vi "Process Controller.vi"() -> ()   [LabVIEW 2015]
doc: "Uses the next generation of Stamp control boxes that have the ability to control pump direction. \n\nAutomatically saves configuration changes to Process Controller.pcm in the same folder as the application.\nKeeps track of whether the program was shutdown correctly with a boolean in the ini file. If the software doesn't shutdown correctly it will automatically resume where it left off (same configuration and same state) as when it was shutdown.\nSaves state name in the state log.\n**********************************\nNo longer reloads setpoint code when not necessary to prevent losing data stored in external code.\nNo longer updates sensor buffer if data wasn't received.\nThe calculated values of setpoints can be viewed \"live\" within the rule editor. This update also adds fields for labeling the output controls. This software can not open the rule files created with previous versions."
uses:
  Plant mode.ctl
  Plant state.ctl
  DAQ configuration/Sensor buffer command.ctl
  file/file action.ctl
  toolbar icons/log data.ctl
  Stamp/calibration commands.ctl
  data status.ctl
  Stamp/stamp command.ctl
  read-write.ctl
  ini interface.ctl
  default or user select.ctl
  toolbar icons/Data Source.ctl
  toolbar icons/peristaltic pump.ctl
  toolbar icons/calibrator.ctl
  toolbar icons/edit rules.ctl
  toolbar icons/Save configuration.ctl
  toolbar icons/open configuration.ctl
  Plant method.ctl
  operator info.ctl
  switch and fraction.ctl
  TCP DAQ/Sensor data.ctl
  DAQ configuration/sensor cluster.ctl
  toolbar icons/file comment.ctl
  toolbar icons/help.ctl
  toolbar icons/Export pcm.ctl
panel:
  in  "Help Button":T1
  out "auto datalogref":refnum<file>
  out "user datalog ref":refnum<file>
  out "TCP ID":refnum<k5>
  in  "Tab Control":T2(tab)=enum."Plant Operation"
  in  "export pcm":T3
  out "data server":string="128.84.245.227"
  out "sensor range error":bool
  in  "Serial Port":refnum<visa-resource-name>="COM1"
  out "Stamp com Failure":bool
  in  "Peristaltic Pump":T4
  in  "Data Source":T5 caption="OK Button"
  in  "Quit":bool
  out "data rate (Hz)":dbl
  out "Datalog File Failure":bool
  in  "Calibrate Sensors":T6
  in  "Edit Rules":T7
  in  "Save":T8
  in  "open":T9
  in  "Process Method":T10={"Operator information"=[], "data log interval"=5, "data loop interval"=20, "Datalog directory path"=path "", "graph update interval"=1.0, "history length"=1000, "Control Logic file path"=path "C:/Documents and Settings/mw24/Desktop/rules.rul", "Sensor Configuration file path"=path "", "HMI VI path"=path "", "HMI data smooth"=0.1} {"HMI data smooth" min=0.01 format="%.2f"; "history length" min=1; "graph update interval" min=0.001 format="%.2f"; "data log interval" min=1}
  out "output descriptions 2":string[][](array[string])
  out "controls 2":T12 {"fractional duty" format="%#_3g"}
  out "Data Status":T13
  out "output descriptions":string[][](array[string])
  in  "Data log interval":sgl=5.0 min=0.01 step=0.01
  in  "Log Data":T14
  in  "File Comment":T15
  out "controls":T12 {"fractional duty" format="%#_3g"}
  in  "Operator Selected State":u16(ring)=1 items=["OFF"]
  out "Elapsed time in current state":dbl format="%.2f"
  out "Process State":u16(ring)=1 items=["OFF"]
  in  "Mode of Operation":T16=enum."Automatic Operation"
  in  "Clear graph":bool
  out "Sensor Data":T17 {"Sensor array"."scaled" format="%.2f"; "Sensor array"."voltage" format="%.4f"; "Time" format="%<%I:%M:%S%2u %p\n%m/%d/%Y>T"}
  out "state graph":cluster{dbl[], dbl[]}(graph)
  in  "sensor to plot":u16(ring) items=["floc interface ()"]
  out "Sensor graph":cluster{dbl[], dbl[]}(graph)
  # "Method files (sensors, rules, calibrations)"
  # "Pump calibration"
  # "Data Source"
  # "Sensor configuration and calibration"
  # "Output communication with Stamp box"
  # "Output:\nstates rules setpoints, controls"
  # "s"
  # "pump off/on"
  # "0"
  # "1"
  # "pump cw/ccw"
  # "1"
  # "pump speed"
  # "2"
  # "pump off/on"
  # "3"
  # "2"
  # "pump cw/ccw"
  # "4"
  # "pump speed"
  # "5"
  # "pump off/on"
  # "6"
  # "3"
  # "pump cw/ccw"
  # "7"
  # "pump speed"
  # "8"
  # "pump off/on"
  # "9"
  # "4"
  # "pump cw/ccw"
  # "10"
  # "pump speed"
  # "11"
  # "pump off/on"
  # "12"
  # "5"
  # "pump cw/ccw"
  # "pump off/on"
  # "0"
  # "pump speed"
  # "pump cw/ccw"
  # "pump speed"
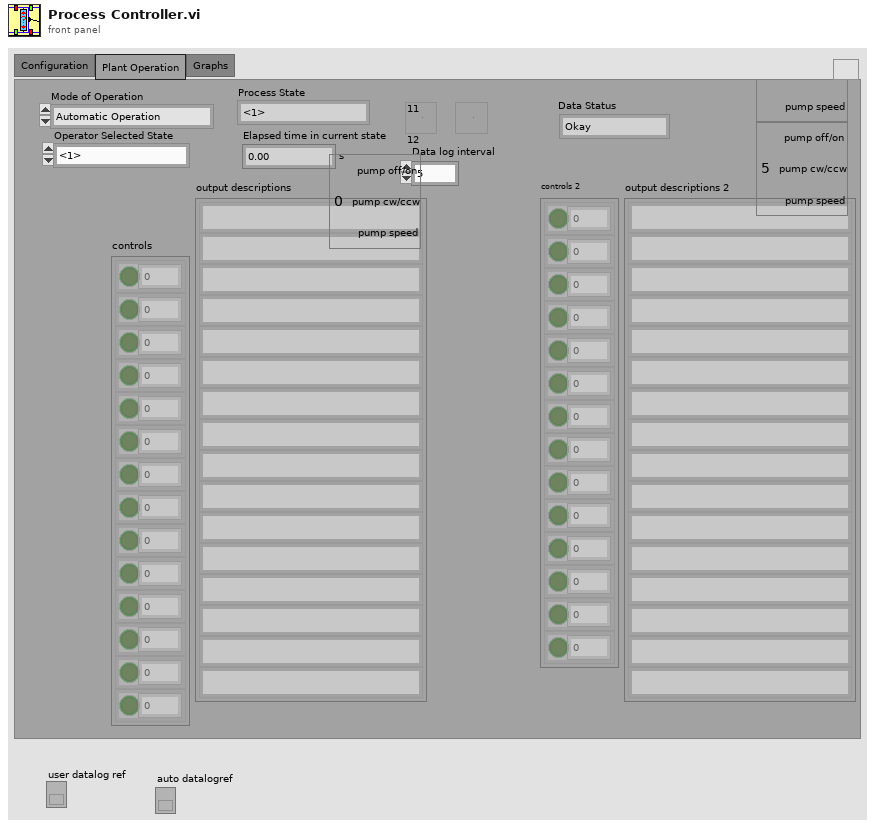
[diagram p1: front panel]
types:
  T1 = typedef "help.ctl" = bool
  T2 = enum32{"Configuration", "Plant Operation", "Graphs"}
  T3 = typedef "Export pcm.ctl" = bool
  T4 = typedef "peristaltic pump.ctl" = bool
  T5 = typedef "Data Source.ctl" = bool
  T6 = typedef "calibrator.ctl" = bool
  T7 = typedef "edit rules.ctl" = bool
  T8 = typedef "Save configuration.ctl" = bool
  T9 = typedef "open configuration.ctl" = bool
  T10 = typedef "Plant method.ctl" = cluster{"Operator information":T11, "data log interval":u32, "data loop interval":u32, "Datalog directory path":path, "graph update interval":sgl, "history length":u16, "Control Logic file path":path, "Sensor Configuration file path":path, "HMI VI path":path, "HMI data smooth":dbl}
  T11 = typedef "operator info.ctl" = cluster{"First name":string, "Last name":string, "NetID":string}[]
  T12 = typedef "switch and fraction.ctl" = cluster{"switch":bool, "fractional duty":dbl}[]
  T13 = typedef "data status.ctl" = enum16{"Okay", "Sensor Range error", "Server error"}
  T14 = typedef "log data.ctl" = bool
  T15 = typedef "file comment.ctl" = bool
  T16 = typedef "Plant mode.ctl" = enum16{"Manual Locked in State", "Automatic Operation"}
  T17 = typedef "Sensor data.ctl" = cluster{" Sensor array":T18[], "Time":dbl}
  T18 = typedef "sensor cluster.ctl" = cluster{"voltage":sgl, "scaled":sgl, "units":string, "Out of Range":bool}
  T19 = typedef "Sensor buffer command.ctl" = enum16{"read average", "read recent", "read all", "write", "set buffer size", "Read channel config", "Write channel config", "clear"}
  T20 = typedef "ini interface.ctl" = enum16{"dataserver list", "dataserver", "com port", "stamp model", "Local Daq"}
  T21 = typedef "read-write.ctl" = enum16{"read", "write"}
  T22 = typedef "calibration commands.ctl" = enum16{"Get ini Path", "Save default values", "Save new calibration", "Read calibration", "Apply calibration", "Read STAMP mb", "Write STAMP mb"}
  T23 = typedef "stamp command.ctl" = enum16{"Configure", "Write", "Off", "Close"}
  T24 = typedef "default or user select.ctl" = enum16{"Default", "User select"}
  T25 = typedef "file action.ctl" = enum16{"Save", "Open"}
  T26 = enum32{"invalid app kind", "Development System", "Run Time System", "Student Edition", "Embedded LabVIEW", "Evaluation", "Custom"}
  T27 = enum16{"open", "open or create", "create or replace", "create", "open (read only)"}
  T28 = typedef "Plant state.ctl" = u16
  T29 = typedef "calibration values.ctl" = cluster{"target 1":dbl[unit], "target 2":dbl[unit], "measured 1":dbl[unit], "measured 2":dbl[unit]}
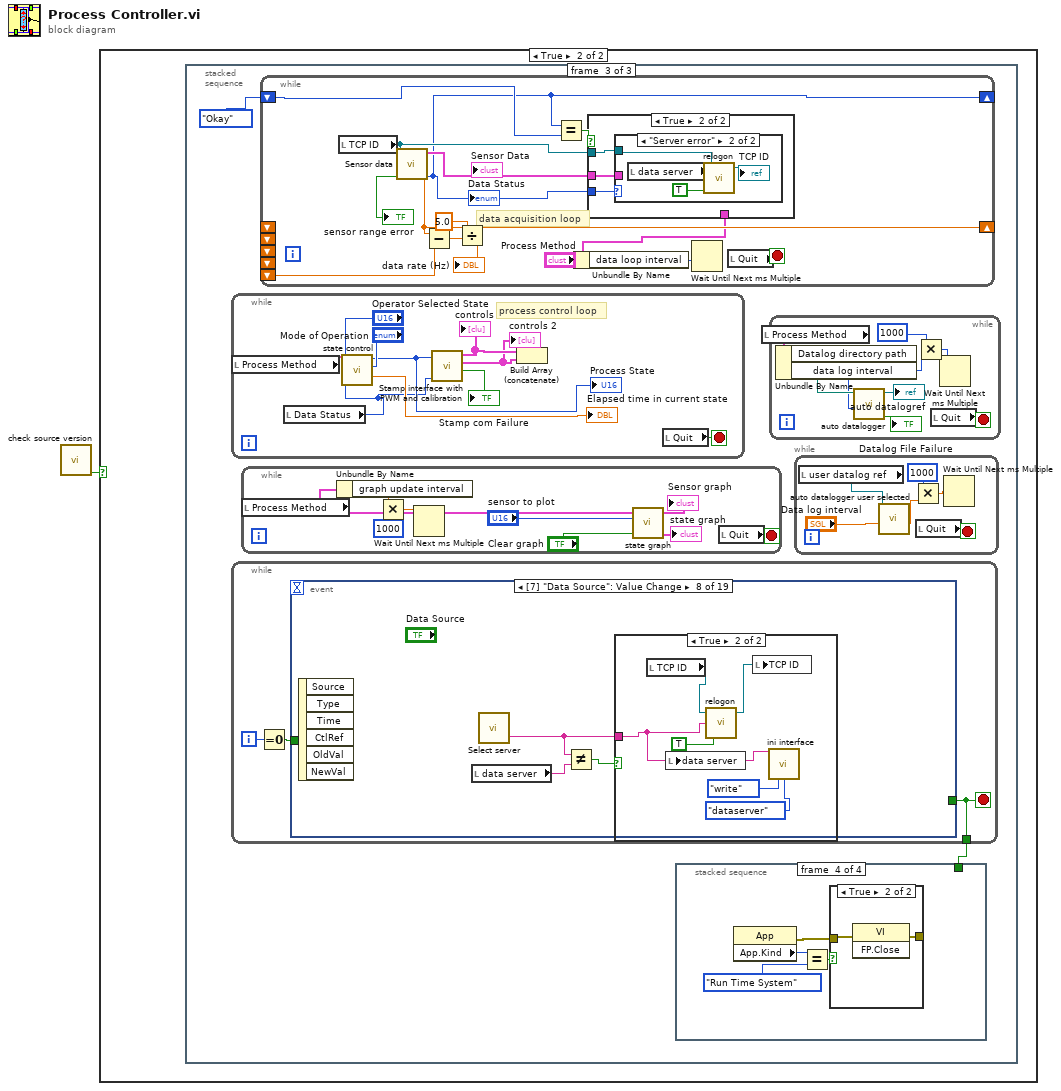
[diagram p0: block diagram]
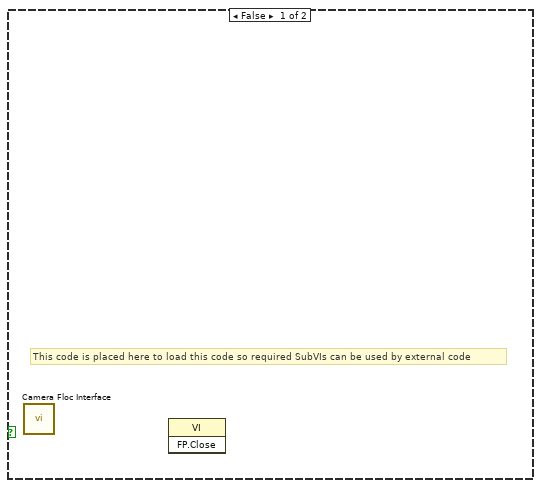
[diagram p2: hidden frame]
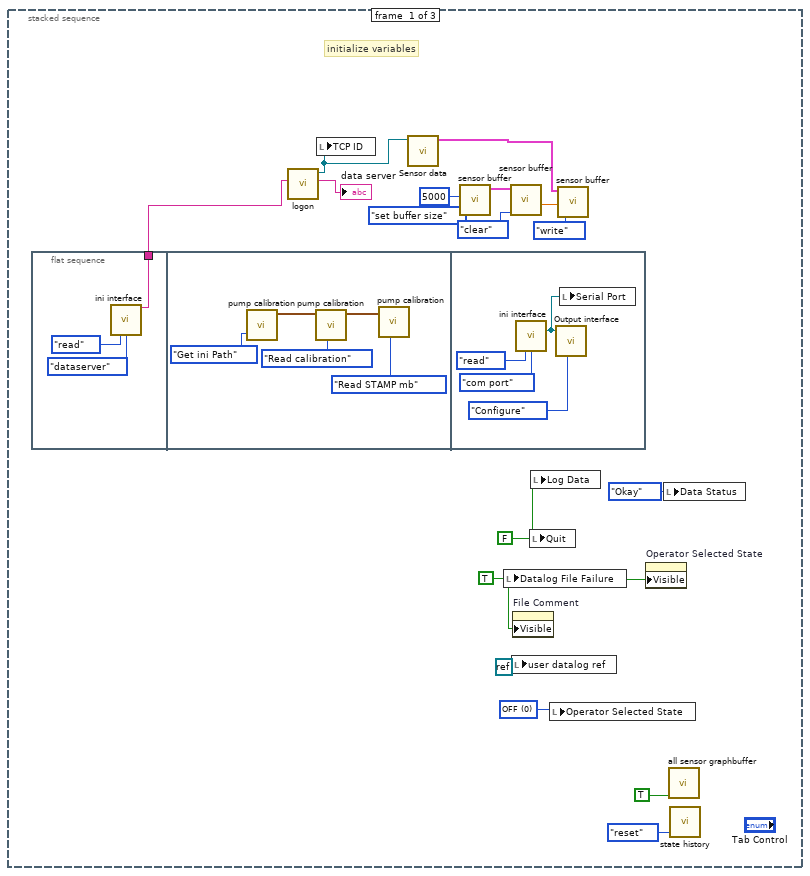
[diagram p3: hidden frame]
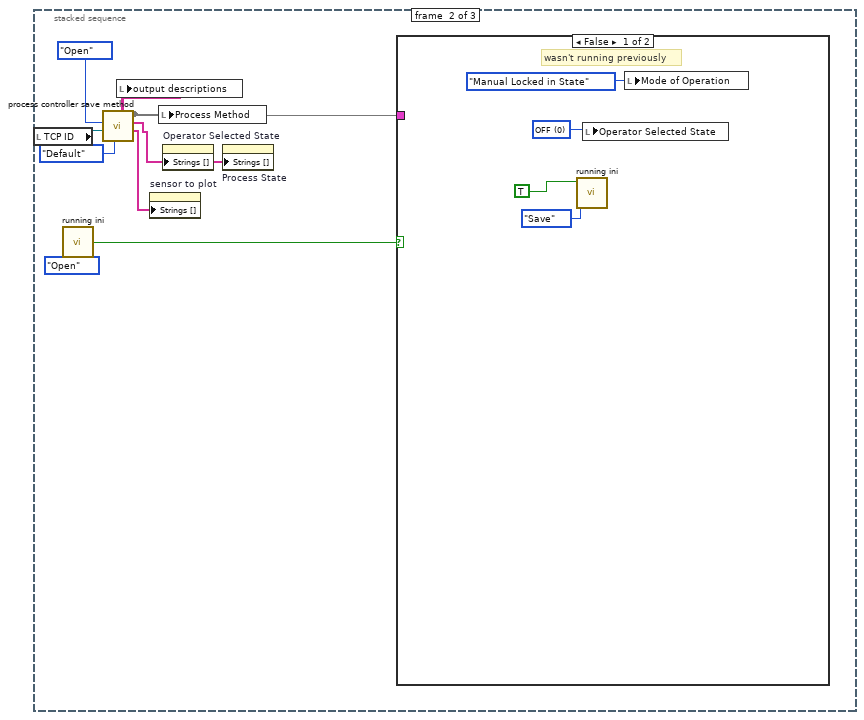
[diagram p4: hidden frame]
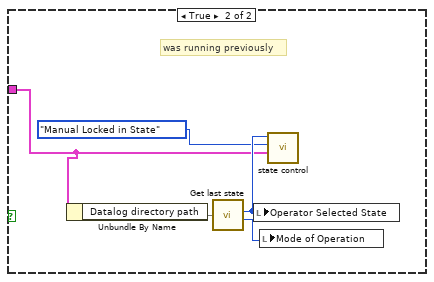
[diagram p5: hidden frame]
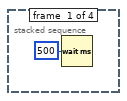
[diagram p6: hidden frame]
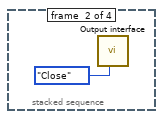
[diagram p7: hidden frame]
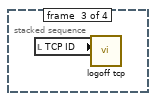
[diagram p8: hidden frame]
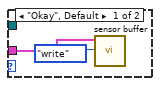
[diagram p11: hidden frame]
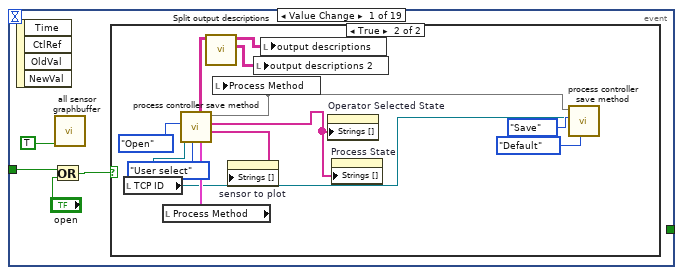
[diagram p12: hidden frame]
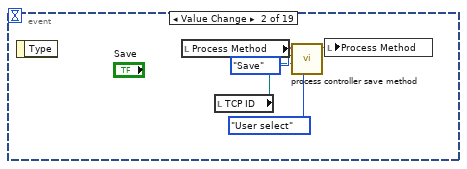
[diagram p14: hidden frame]
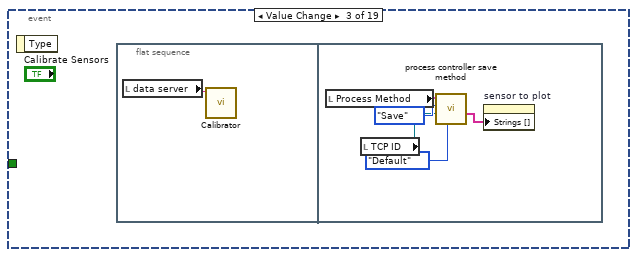
[diagram p15: hidden frame]
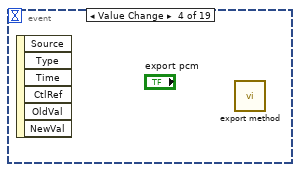
[diagram p16: hidden frame]
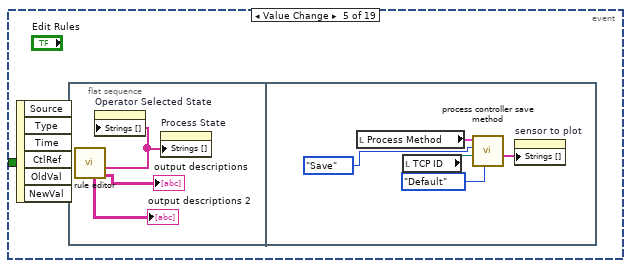
[diagram p17: hidden frame]
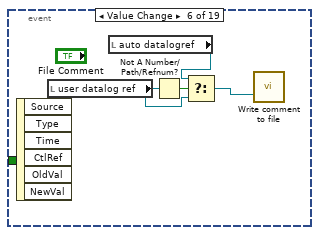
[diagram p18: hidden frame]
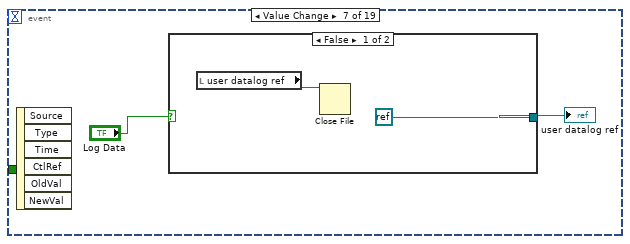
[diagram p19: hidden frame]
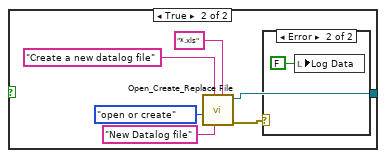
[diagram p20: hidden frame]
diagram:
  n1 = call "check source version.vi"() -> ("continue running?"=w1:bool)  [unwired: 4 in, 1 out]
  n2 = case shown="True" w1 {
    frame False {
      # "This code is placed here to load this code so required SubVIs can be used by external code"
      n3 = call "Camera Floc Interface.vi"() -> ()  [unwired: 6 in, 2 out]
      n4 = invoke class="VI" method="FP.Close"() -> ()  [unwired: 3 in, 3 out]
    }
    frame True {
      n5 = stacked-sequence {
        frame #0 {
          w10 = T28 0 items=["OFF"] ("Operator Selected State")
          w2 = TRUE ("stop")
          w11 = FALSE ("stop")
          # "initialize variables"
          n6 = flat-sequence {
            tunnel: [w19] -> w3
            frame #0 {
              n7 = call "ini interface.vi"("direction"=read-write."read", "ini interface"=ini_interface."dataserver") -> ("dataserver out"=w19:string)  [unwired: 9 in, 4 out]
            }
            frame #1 {
              n8 = call "pump calibration.vi"("pump cal command"=calibration_commands."Get ini Path") -> ("Pump Calibration out"=w23:T29)  [unwired: 7 in, 3 out]
              n9 = call "pump calibration.vi"("pump cal command"=calibration_commands."Read calibration", "Pump Calibration in"=w23) -> ("Pump Calibration out"=w26:T29)  [unwired: 6 in, 3 out]
              n10 = call "pump calibration.vi"("pump cal command"=calibration_commands."Read STAMP mb", "Pump Calibration in"=w26) -> ()  [unwired: 6 in, 4 out]
            }
            frame #2 {
              n11 = call "ini interface.vi"("direction"=read-write."read", "ini interface"=ini_interface."com port") -> ("Serial Port out"=w30:refnum<visa-resource-name>)  [unwired: 9 in, 4 out]
              n12 = call "Output interface.vi"("Stamp Command"=stamp_command."Configure", "DeviceName"=w30) -> ()  [unwired: 8 in, 2 out]
              n13 = local write "Serial Port"(w30) -> ()
            }
          }
          n14 = call "logon.vi"("data server address in"=w3) -> ("data server address"=→"data server":string, "connection ID"=w9:refnum<k5>)  [unwired: 7 in, 2 out]
          n15 = local write "TCP ID"(w9) -> ()
          n16 = call "Sensor data.vi"("Connection ID in"=w9) -> ("Sensor Data"=w6:T17)  [unwired: 3 in, 7 out]
          n17 = call "sensor buffer.vi"("command"=Sensor_buffer_command."set buffer size", "max array size"=u16 5000) -> ("Sensor Data smoothed"=w8:T17)  [unwired: 3 in, 2 out]
          n18 = local write "Datalog File Failure"(w2) -> ()
          n19 = call "sensor buffer.vi"("command"=Sensor_buffer_command."clear", "Sensor Data"=w8) -> ("data rate (Hz)"=w5:sgl)  [unwired: 3 in, 2 out]
          n20 = local write "user datalog ref"(refnum<k0> refnum) -> ()
          n21 = property on="File Comment" class="Bool"("Visible"=w2) -> ()  [unwired: 2 in, 2 out]
          n22 = local write "Quit"(w11) -> ()
          n23 = local write "Log Data"(w11) -> ()
          n24 = local write "Operator Selected State"(w10) -> ()
          n25 = call "sensor buffer.vi"("command"=Sensor_buffer_command."write", "smooth interval (s)"=w5, "Sensor Data"=w6) -> ()  [unwired: 2 in, 3 out]
          n26 = property on="Operator Selected State" class="Ring (strict)"("Visible"=w2) -> ()  [unwired: 2 in, 2 out]
          n27 = local write "Data Status"(data_status."Okay" ("Data Status")) -> ()
          n28 = call "all sensor graphbuffer.vi"("Reset"=TRUE) -> ()  [unwired: 8 in, 3 out]
          n29 = call "state history.vi"("command"=enum16{"write", "read", "reset"}."reset") -> ()  [unwired: 2 in, 1 out]
        }
        frame #1 {
          n30 = local read "TCP ID"() -> (w32:refnum<k5>)
          n31 = call "running ini.vi"("Action"=file_action."Open") -> ("running out"=w38:bool)  [unwired: 5 in]
          n32 = call "process controller save method.vi"("default or user"=default_or_user_select."Default", 9:w32, "Action"=file_action."Open") -> ("sensor &var names"=w37:string[], "State names"=w35:string[], 3:w34, "output descriptions out"=w36:string[][])  [unwired: 4 in, 1 out]
          n33 = local write "output descriptions"(w36) -> ()
          n34 = property on="sensor to plot" class="Ring (strict)"("Strings []"=w37) -> ()  [unwired: 2 in, 2 out]
          n35 = local write "Process Method"(w34) -> ()
          n36 = property on="Operator Selected State" class="Ring (strict)"("Strings []"=w35) -> ()  [unwired: 2 in, 2 out]
          n37 = property on="Process State" class="Ring (strict)"("Strings []"=w35) -> ()  [unwired: 2 in, 2 out]
          n38 = case shown="False" w38 {
            tunnel: w34 -> [_ w45]
            frame False {
              w40 = T28 0 items=["OFF"] ("Operator Selected State")
              # "wasn't running previously"
              n39 = call "running ini.vi"("running in"=TRUE ("running"), "Action"=file_action."Save") -> ()  [unwired: 4 in, 1 out]
              n40 = local write "Operator Selected State"(w40) -> ()
              n41 = local write "Mode of Operation"(Plant_mode."Manual Locked in State" ("Plant Mode of Operation")) -> ()
            }
            frame True {
              # "was running previously"
              n42 = Unbundle By Name(w45) -> ("Datalog directory path"=w48)
              n43 = call "Get last state.vi"("Datalog directory path"=w48) -> ("Plant State"=w47:T28, "Plant Mode of Operation"=w44:T16)  [unwired: 2 in]
              n44 = local write "Operator Selected State"(w47) -> ()
              n45 = local write "Mode of Operation"(w44) -> ()
              n46 = call "state control.vi"("Datalog directory path"=w45, "Plant Mode of Operation"=Plant_mode."Manual Locked in State", "Operator Selected State"=w47) -> ()  [unwired: 6 in, 3 out]
            }
          }
        }
        frame #2 {
          n47 = while {
            stop <- w92 stop-if-true
            # "process control loop"
            n48 = local read "Process Method"() -> (w89:T10)
            n49 = local read "Data Status"() -> (w86:T13)
            n50 = call "state control.vi"(8:w86, "Datalog directory path"=w89, "Plant Mode of Operation"="Mode of Operation", "Operator Selected State"="Operator Selected State") -> ("Elapsed time in current state"=→"Elapsed time in current state":dbl, "Plant State out"=w87:u16)  [unwired: 5 in, 1 out]
            "Process State" <- w87
            n51 = call "Stamp interface with PWM and calibration.vi"("error in"=w86, "Plant State"=w87) -> ("NI board success"=→"Stamp com Failure":bool, "Variables"=w83:cluster{string, "value":dbl}[], "Controls out 1"=w84:T12)  [unwired: 6 in, 1 out]
            "controls" <- w84
            "controls 2" <- w83
            n52 = Build Array (concatenate)(w84, w83) -> ()  [unwired: 1 out]
            n53 = local read "Quit"() -> (w92:bool)
          }
          n54 = while {
            tunnel: [w116] -> w50
            i -> [w117]
            stop <- w116 stop-if-true
            n55 = Equal To 0?(x=w117) -> (x = 0?=w118:bool)
            n56 = event shown="[7] \"Data Source\": Value Change" {
              selector: _ -> [_ _ _ _ _ _ _ _ _ _ _ _ _ _ _ _ _ _ _]
              dyn-events: _ -> [_ _ _ _ _ _ _ _ _ _ _ _ _ _ _ _ _ _ _]
              timeout: _ -> [_ _ _ _ _ _ _ _ _ _ _ _ _ _ _ _ _ _ _]
              tunnel: w118 -> [w120 _ _ _ _ _ _ _ _ _ _ _ _ _ _ _ _ _ _]
              tunnel: [_ _ _ _ _ _ _ _ _ _ _ _ _ _ _ "Quit" w210 w213 _] -> w116
              event Value Change {
                n57 = event-data() -> ()  [unwired: 1 in, 4 out]
                n58 = Or(x=w120, y="open") -> (x .or. y?=w119:T9)
                n59 = call "all sensor graphbuffer.vi"("Reset"=TRUE) -> ()  [unwired: 8 in, 3 out]
                n60 = case shown="True" w119 {
                  frame False {
                  }
                  frame True {
                    n61 = local read "TCP ID"() -> (w128:refnum<k5>)
                    n62 = local read "Process Method"() -> (w132:T10)
                    n63 = call "process controller save method.vi"("default or user"=default_or_user_select."User select", 9:w128, "Action"=file_action."Open", 11:w132) -> ("sensor &var names"=w133:string[], "State names"=w131:string[], 3:w129, "output descriptions out"=w125:string[][])  [unwired: 3 in, 1 out]
                    n64 = call "Split output descriptions.vi"("output descriptions combined"=w125) -> ("output descriptions 2"=w123:string[][], "output descriptions"=w124:string[][])  [unwired: 9 in]
                    n65 = local write "Process Method"(w129) -> ()
                    n66 = property on="sensor to plot" class="Ring (strict)"("Strings []"=w133) -> ()  [unwired: 2 in, 2 out]
                    n67 = local write "output descriptions 2"(w123) -> ()
                    n68 = local write "output descriptions"(w124) -> ()
                    n69 = property on="Operator Selected State" class="Ring (strict)"("Strings []"=w131) -> ()  [unwired: 2 in, 2 out]
                    n70 = property on="Process State" class="Ring (strict)"("Strings []"=w131) -> ()  [unwired: 2 in, 2 out]
                    n71 = call "process controller save method.vi"("default or user"=default_or_user_select."Default", 9:w128, "Action"=file_action."Save", 11:w129) -> ()  [unwired: 4 in, 4 out]
                  }
                }
              }
              event Value Change {
                n72 = event-data() -> ()  [unwired: 1 in, 1 out]
                n73 = local read "Process Method"() -> (w137:T10)
                n74 = local read "TCP ID"() -> (w136:refnum<k5>)
                n75 = call "process controller save method.vi"("default or user"=default_or_user_select."User select", 9:w136, "Action"=file_action."Save", 11:w137) -> (3:w138)  [unwired: 3 in, 4 out]
                n76 = local write "Process Method"(w138) -> ()
              }
              event Value Change {
                n77 = event-data() -> ()  [unwired: 1 in, 1 out]
                n78 = flat-sequence {
                  frame #0 {
                    n79 = local read "data server"() -> (w140:string)
                    n80 = call "Calibrator.vi"(0:w140) -> ()  [unwired: 8 in, 2 out]
                  }
                  frame #1 {
                    n81 = local read "Process Method"() -> (w144:T10)
                    n82 = local read "TCP ID"() -> (w143:refnum<k5>)
                    n83 = call "process controller save method.vi"("default or user"=default_or_user_select."Default", 9:w143, "Action"=file_action."Save", 11:w144) -> ("sensor &var names"=w142:string[])  [unwired: 4 in, 3 out]
                    n84 = property on="sensor to plot" class="Ring (strict)"("Strings []"=w142) -> ()  [unwired: 2 in, 2 out]
                  }
                }
              }
              event Value Change {
                n85 = event-data() -> ()  [unwired: 1 in, 6 out]
                n86 = call "export method.vi"() -> ()  [unwired: 1 in]
              }
              event Value Change {
                n87 = event-data() -> ()  [unwired: 1 in, 6 out]
                n88 = flat-sequence {
                  frame #0 {
                    n89 = call "rule editor.vi"() -> ("output descriptions out"=→"output descriptions":string[][], "State names"=w147:string[], "output descriptions out 2"=→"output descriptions 2":string[][])  [unwired: 8 in, 1 out]
                    n90 = property on="Operator Selected State" class="Ring (strict)"("Strings []"=w147) -> ()  [unwired: 2 in, 2 out]
                    n91 = property on="Process State" class="Ring (strict)"("Strings []"=w147) -> ()  [unwired: 2 in, 2 out]
                  }
                  frame #1 {
                    n92 = local read "Process Method"() -> (w152:T10)
                    n93 = local read "TCP ID"() -> (w151:refnum<k5>)
                    n94 = call "process controller save method.vi"("default or user"=default_or_user_select."Default", 9:w151, "Action"=file_action."Save", 11:w152) -> ("sensor &var names"=w150:string[])  [unwired: 4 in, 3 out]
                    n95 = property on="sensor to plot" class="Ring (strict)"("Strings []"=w150) -> ()  [unwired: 2 in, 2 out]
                  }
                }
              }
              event Value Change {
                n96 = event-data() -> ()  [unwired: 1 in, 6 out]
                n97 = local read "user datalog ref"() -> (w155:refnum<file>)
                n98 = local read "auto datalogref"() -> (w154:refnum<file>)
                n99 = Not A Number/Path/Refnum?(number/path/refnum=w155) -> (NaN/Path/Refnum?=w157:bool)
                n100 = Select(t=w154, s=w157, f=w155) -> (s? t:f=w156:refnum<file>)
                n101 = call "Write comment to file.vi"("refnum"=w156) -> ()  [unwired: 7 in, 2 out]
              }
              event Value Change {
                n102 = event-data() -> ()  [unwired: 1 in, 6 out]
                n103 = case shown="False" "Log Data" {
                  tunnel: [refnum<k0> refnum w164] -> w159
                  frame False {
                    n104 = local read "user datalog ref"() -> (w161:refnum<file>)
                    n105 = Close File(refnum=w161) -> ()  [unwired: 1 in, 2 out]
                  }
                  frame True {
                    n106 = call <vilib>:"Open_Create_Replace File.vi"("pattern"="*.xls", "default name"="New Datalog file", "prompt"="Create a new datalog file", "function (open:0)"=T27."open or create") -> ("error out"=w162:errorcluster, "refnum"=w164:refnum<file>)  [unwired: 4 in, 2 out]
                    n107 = case shown="Error" w162 {
                      frame No Error {
                      }
                      frame Error {
                        n108 = local write "Log Data"(T14 FALSE ("Log Data")) -> ()
                      }
                    }
                  }
                }
                "user datalog ref" <- w159
              }
              event Value Change {
                n109 = event-data() -> ()  [unwired: 1 in, 6 out]
                n110 = local read "data server"() -> (w170:string)
                n111 = call "Select server.vi"() -> ("DataSource"=w171:string)  [unwired: 5 in]
                n112 = Not Equal?(x=w171, y=w170) -> (x != y?=w169:bool)
                n113 = case shown="True" w169 {
                  tunnel: w171 -> [_ w174]
                  frame False {
                  }
                  frame True {
                    n114 = local read "TCP ID"() -> (w175:refnum<k5>)
                    n115 = local write "data server"(w174) -> ()
                    n116 = call "relogon.vi"("relogon"=TRUE, "data server address in"=w174, "Connection ID"=w175) -> ("connection ID out"=w172:refnum<k5>)  [unwired: 2 in]
                    n117 = local write "TCP ID"(w172) -> ()
                    n118 = call "ini interface.vi"("dataserver"=w174, "direction"=read-write."write", "ini interface"=ini_interface."dataserver") -> ()  [unwired: 8 in, 5 out]
                  }
                }
              }
              event Value Change {
                n119 = event-data() -> ()  [unwired: 1 in, 6 out]
                n120 = call "Application name.vi"() -> ("help site"=w178:string)  [unwired: 5 in, 2 out]
                n121 = call "Web Browser.vi"("URL"=w178) -> ()  [unwired: 1 in]
              }
              event "Serial Port": Value Change {
                n122 = event-data() -> ()  [unwired: 1 in, 6 out]
                n123 = call "Output interface.vi"("Stamp Command"=stamp_command."Configure", "DeviceName"="Serial Port") -> ()  [unwired: 8 in, 2 out]
                n124 = call "ini interface.vi"("Serial Port"="Serial Port", "direction"=read-write."write", "ini interface"=ini_interface."com port") -> ()  [unwired: 8 in, 5 out]
              }
              event "Clear graph": Value Change {
                n125 = event-data() -> ()  [unwired: 1 in, 5 out]
                n126 = call "state history.vi"("command"=enum16{"write", "read", "reset"}."reset") -> ()  [unwired: 2 in, 1 out]
              }
              event "sensor to plot": Value Change; "sensor to plot": Mouse Down {
                n127 = event-data() -> ()  [unwired: 1 in, 3 out]
                n128 = local read "sensor to plot"() -> (w185:u16)
                n129 = property on="sensor to plot" class="Ring (strict)"() -> ("Strings []"=w188:string[])  [unwired: 2 in, 2 out]
                n130 = Index Array(array=w188, index=w185) -> (element=w186:string)
                n131 = Build Array(w185) -> (w184:u16[])
                n132 = property on="Sensor graph" class="XYGraph (strict)"("Active Y Scale"=u32 0 ("Active Plot"), "Y Scale.Name Label.Text"=w186) -> ()  [unwired: 2 in, 2 out]
                n133 = property on="Sensor array" class="Arr (strict)"("Index Values"=w184) -> ()  [unwired: 2 in, 2 out]
              }
              event Value Change {
                n134 = event-data() -> ("NewVal"=w199:path)  [unwired: 1 in, 5 out]
                n135 = Strip Path(path=w199) -> (stripped path=w198:path)  [unwired: 1 out]
                n136 = File/Directory Info(path=w199) -> (directory=w200:bool)  [unwired: 1 in, 6 out]
                n137 = Select(t=w199, s=w200, f=w198) -> (s? t:f=w195:path)
                n138 = local read "Process Method"() -> (w202:T10)
                n139 = Not A Number/Path/Refnum?(number/path/refnum=w195) -> (NaN/Path/Refnum?=w193:bool)
                n140 = Empty String/Path?(string/path=w195) -> (empty?=w192:bool)
                n141 = Bundle By Name(cluster=w202, "Datalog directory path"=w195) -> (w201:T10)
                n142 = File/Directory Info(path=w195) -> (directory=w196:bool)  [unwired: 1 in, 6 out]
                n143 = Not(x=w196) -> (.not. x?=w194:bool)
                n144 = Compound Arithmetic op=OR(w194, w193, w192) -> (invert w190:bool)
                n145 = local read "Log Data"() -> (w191:T14)
                n146 = Not(x=w190) -> (.not. x?=w197:bool)
                n147 = Or(x=w190, y=w191) -> (x .or. y?=w189:T14)
                n148 = local write "Datalog File Failure"(w197) -> ()
                n149 = property on="File Comment" class="Bool"("Visible"=w189) -> ()  [unwired: 2 in, 2 out]
                n150 = local write "Process Method"(w201) -> ()
              }
              event Value Change {
                n151 = event-data() -> ("NewVal"=w205:T10)  [unwired: 1 in, 5 out]
                n152 = local read "TCP ID"() -> (w204:refnum<k5>)
                n153 = call "process controller save method.vi"("default or user"=default_or_user_select."Default", 9:w204, "Action"=file_action."Save", 11:w205) -> ()  [unwired: 4 in, 4 out]
              }
              event Value Change {
                n154 = event-data() -> ()  [unwired: 1 in, 6 out]
                n155 = call "pump calibration dialog.vi"() -> ()  [unwired: 1 in]
              }
              event "Quit": Value Change; Panel Close {
                (unwired) TRUE ("Quit")
                # "This is a normal (user initiated) shutdown."
                n156 = event-data() -> ()  [unwired: 1 in, 2 out]
                n157 = call "running ini.vi"("running in"=FALSE ("running"), "Action"=file_action."Save") -> ()  [unwired: 4 in, 1 out]
              }
              event Panel Close? {
                w210 = TRUE ("Quit")
                # "This is a normal (user initiated) shutdown."
                n158 = event-data() -> ()  [unwired: 1 in, 4 out]
                n159 = call "running ini.vi"("running in"=FALSE ("running"), "Action"=file_action."Save") -> ()  [unwired: 4 in, 1 out]
                n160 = local write "Quit"(w210) -> ()
                n161 = event-data("Discard?"=w210) -> ()  [unwired: 1 in, 1 out]
              }
              event Application Instance Close? {
                w213 = TRUE ("Quit")
                n162 = event-data() -> ()  [unwired: 1 in, 5 out]
                n163 = local write "Quit"(w213) -> ()
                n164 = event-data("Discard?"=w213) -> ()  [unwired: 2 in, 1 out]
              }
              event "Operator Selected State": Value Change; "Operator Selected State": Mouse Up {
                n165 = event-data() -> ()  [unwired: 1 in, 3 out]
                n166 = local read "Operator Selected State"() -> (w214:u16)
                n167 = local read "Process Method"() -> (w216:T10)
                n168 = call "state control.vi"("Datalog directory path"=w216, "Plant Mode of Operation"=Plant_mode."Manual Locked in State", "Operator Selected State"=w214) -> ()  [unwired: 6 in, 3 out]
              }
            }
          }
          n169 = while {
            stop <- w80 stop-if-true
            n170 = local read "Process Method"() -> (w74:T10)
            n171 = Unbundle By Name(w74) -> ("graph update interval"=w79:sgl)
            n172 = Multiply(x=w79, y=i16 1000) -> (x*y=w81:sgl)
            n173 = Wait Until Next ms Multiple(millisecond multiple=w81) -> ()  [unwired: 1 out]
            n174 = call "state graph.vi"("Clear graph"="Clear graph", "sensor to plot"="sensor to plot", "Plant Method"=w74) -> ("state graph"=→"state graph":cluster{dbl[], dbl[]}, "sensor graph"=→"Sensor graph":cluster{dbl[], dbl[]})  [unwired: 1 out]
            n175 = local read "Quit"() -> (w80:bool)
          }
          n176 = while {
            shift-right: [w104] -> _
            shift-left: _ -> [_]
            shift-left: _ -> [_]
            shift-left: _ -> [_]
            shift-left: _ -> [_]
            shift-left: _ -> [w103]
            shift-right: [w93] -> _
            shift-left: data_status."Okay" ("Data Status") -> [w96]
            stop <- w106 stop-if-true
            # "data acquisition loop"
            n177 = local read "TCP ID"() -> (w99:refnum<k5>)
            n178 = call "Sensor data.vi"("Connection ID in"=w99) -> ("Data Status"=w93:T13, "time (s)"=w104:dbl, "Sensor Data"=w98:T17, "sensor range error"=→"sensor range error":bool)  [unwired: 3 in, 4 out]
            "Sensor Data" <- w98
            "Data Status" <- w93
            n179 = Subtract(x=w104, y=w103) -> (x-y=w102:dbl)
            n180 = Divide(x=5.0, y=w102) -> (x/y=→"data rate (Hz)":dbl)
            n181 = Equal?(x=w93, y=w96) -> (x = y?=w97:bool)
            n182 = Unbundle By Name("Process Method") -> ("data loop interval"=w105:u32)
            n183 = case shown="True" w97 {
              tunnel: w99 -> [_ w109]
              tunnel: w98 -> [_ w108]
              tunnel: w93 -> [_ w107]
              tunnel: "Process Method" -> [_ _]
              frame False {
              }
              frame True {
                n184 = case shown="\"Server error\"" w107 {
                  tunnel: w109 -> [_ w115]
                  tunnel: w108 -> [w111 _]
                  frame "Okay", Default {
                    n185 = call "sensor buffer.vi"("command"=Sensor_buffer_command."write", "Sensor Data"=w111) -> ()  [unwired: 3 in, 3 out]
                  }
                  frame "Server error" {
                    n186 = local read "data server"() -> (w113:string)
                    n187 = call "relogon.vi"("relogon"=TRUE, "data server address in"=w113, "Connection ID"=w115) -> ("connection ID out"=→"TCP ID":refnum<k5>)  [unwired: 2 in]
                  }
                }
              }
            }
            n188 = Wait Until Next ms Multiple(millisecond multiple=w105) -> ()  [unwired: 1 out]
            n189 = local read "Quit"() -> (w106:bool)
          }
          n190 = stacked-sequence {
            tunnel: w50 -> [_ _ _ _]
            frame #0 {
              n191 = Wait (ms)(milliseconds to wait=u32 500) -> ()  [unwired: 1 out]
            }
            frame #1 {
              n192 = call "Output interface.vi"("Stamp Command"=stamp_command."Close") -> ()  [unwired: 9 in, 2 out]
            }
            frame #2 {
              n193 = local read "TCP ID"() -> (w53:refnum<k5>)
              n194 = call "logoff tcp.vi"("Connection ID"=w53) -> ()  [unwired: 9 in, 2 out]
            }
            frame #3 {
              n195 = property class="App"() -> (error out=w57:errorcluster, "App.Kind"=w55:T26)  [unwired: 2 in, 1 out]
              n196 = Equal?(x=w55, y=T26."Run Time System" ("Application:Kind")) -> (x = y?=w56:bool)
              n197 = case shown="True" w56 {
                tunnel: w57 -> [w58 w60]
                tunnel: [w58 w59] -> _
                frame False {
                }
                frame True {
                  n198 = invoke class="VI" method="FP.Close"(error in=w60) -> (error out=w59:errorcluster)  [unwired: 2 in, 2 out]
                }
              }
            }
          }
          n199 = while {
            stop <- w72 stop-if-true
            n200 = local read "Process Method"() -> (w73:T10)
            n201 = Unbundle By Name(w73) -> ("Datalog directory path"=w71:path, "data log interval"=w67:u32)
            n202 = call "auto datalogger.vi"("data log interval (s)"=w67, "Datalog directory path"=w71) -> ("File Failure"=→"Datalog File Failure":bool, "File refnum"=→"auto datalogref":refnum<file>)  [unwired: 8 in]
            n203 = Multiply(x=i16 1000 ("y"), y=w67) -> (x*y=w68:u32)
            n204 = local read "Quit"() -> (w72:bool)
            n205 = Wait Until Next ms Multiple(millisecond multiple=w68) -> ()  [unwired: 1 out]
          }
          n206 = while {
            stop <- w65 stop-if-true
            n207 = local read "user datalog ref"() -> (w62:refnum<file>)
            n208 = call "auto datalogger user selected.vi"("data log interval (s)"="Data log interval", "datalog ref"=w62) -> ()  [unwired: 8 in, 2 out]
            n209 = Multiply(x=i16 1000 ("y"), y="Data log interval") -> (x*y=w63:sgl)
            n210 = local read "Quit"() -> (w65:bool)
            n211 = Wait Until Next ms Multiple(millisecond multiple=w63) -> ()  [unwired: 1 out]
          }
        }
      }
    }
  }
